vi "RSZVB Set Permanent Signal Source State.vi"(7 "State (F: Off)":bool, 8 "error in (no error)":errorcluster {"code" format="%.0x"}, 9 "Port (1)":i32=1, 10 "Channel (1)":i32=1, 11 "VISA session":refnum<visa-resource-name>) -> (0 "error out":errorcluster {"code" format="%.0x"}, 3 "dup VISA session":refnum<visa-resource-name>)   [LabVIEW 2011]
doc: "This VI defines whether the source power is permanently on. \n\nRemote-control command(s):\nSOURce<Ch>:POWer<Pt>:PERManent[:STATe] <Boolean>"
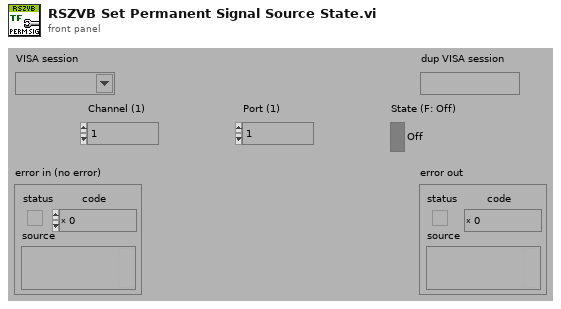
[diagram p1: front panel]
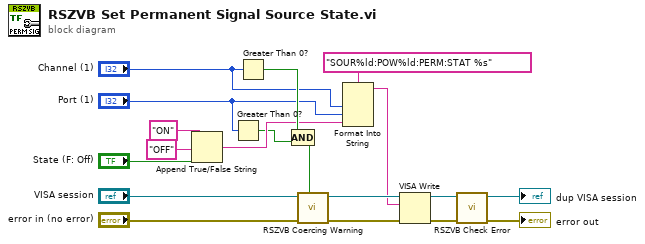
[diagram p0: block diagram]
diagram:
  n1 = Append True/False String(1:"State (F: Off)", 2:"OFF", 3:"ON") -> (0:w9:string)  [unwired: 1 in]
  n2 = Greater Than 0?(x="Port (1)") -> (x > 0?=w8:bool)
  n3 = Greater Than 0?(x="Channel (1)") -> (x > 0?=w12:bool)
  n4 = Compound Arithmetic op=AND(w12, w8) -> (w14:bool)
  n5 = call "RSZVB Coercing Warning.vi"("In Range?"=w14, "error in (no error)"="error in (no error)", "VISA session"="VISA session") -> ("error out"=w17:errorcluster, "dup VISA session"=w18:refnum<visa-resource-name>)  [unwired: 7 in]
  n6 = Format Into String(format string="SOUR%ld:POW%ld:PERM:STAT %s", "Channel (1)", "Port (1)", w9) -> (resulting string=w13:string)  [unwired: 2 in, 1 out]
  n7 = VISA Write(VISA resource name=w18, write buffer=w13, error in (no error)=w17) -> (VISA resource name out=w15:refnum<visa-resource-name>, error out=w16:errorcluster)  [unwired: 1 out]
  n8 = call "RSZVB Check Error.vi"("error in (no error)"=w16, "VISA session"=w15) -> ("error out"=→"error out":errorcluster, "dup VISA session"=→"dup VISA session":refnum<visa-resource-name>)  [unwired: 8 in]
